vi "Edit.Path.TestLauncher.vi"() -> ()   [LabVIEW 2019, in "Edit.Path.lvclass"]
uses:
  Edit.Path.lvclass
  <vilib>/JKI/JKI SMO/SMO/Typedefs/SMOState --Enum.ctl
  C:/Program Files (x86)/National Instruments/LabVIEW 2019/vi.lib/JKI/JKI SMO/SMO/SMO.lvclass
  C:/Users/Albro/Documents/GitHub/AFM-Lithography/lvsrc/Classes/Subpanel/Edit/Edit/Edit.lvclass
  <vilib>/JKI/JKI SMO/SMO/SMO.lvclass/SMO.ctl
  <vilib>/JKI/JKI SMO/SMO/Private/ReftoDVR--SMO.vi
  <vilib>/JKI/JKI SMO/SMO/SMO.lvclass
  Edit/Edit.lvclass
panel:
  out "SMO State":T1
  out "error out":errorcluster
  in  "Stop":bool
  # "Basic SMO Test Launcher"
  # "For instructions on how to use the JKI State Machine Objects, examples and video tutorials, visit:\nhttp://jki.net/state-machine-objects/\n\nJKI State Machine Objects™\nhttp://jki.net/state-machine-objects/\nCopyright (C) 2005-2015, JKI <info@jki.net>\nALL RIGHTS RESERVED"
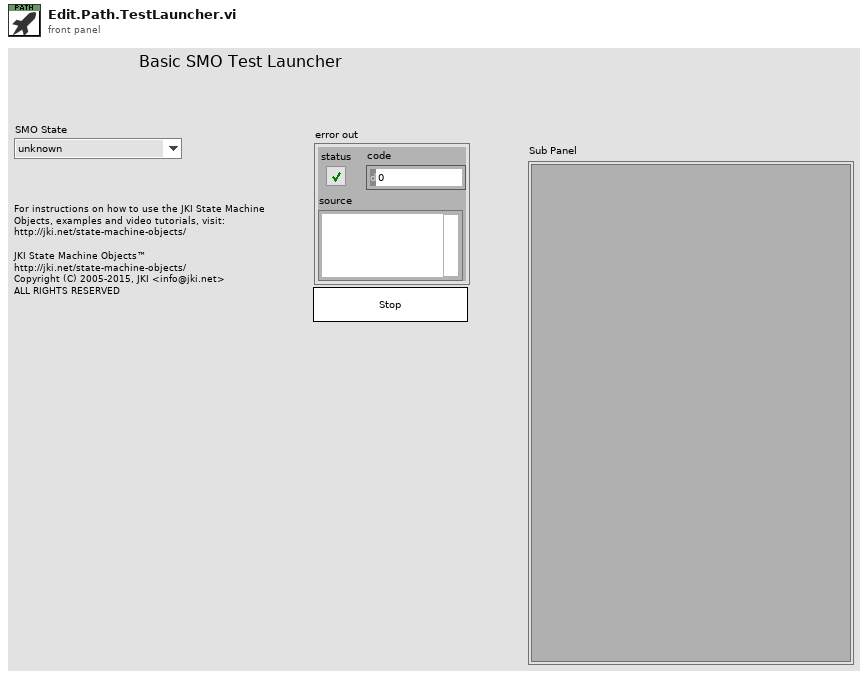
[diagram p1: front panel]
types:
  T1 = typedef "SMO.lvclass/SMOState --Enum.ctl" = enum16{"unknown", "Created", "Started", "Stopped"}
  T2 = typedef "SMO.lvclass/Public Events.ctl" = cluster{"Error":refnum<user-event>, "State":refnum<user-event>, "Reserve State":refnum<user-event>}
  T3 = cluster{"Event Registration Refnum":refnum<event-registration>}
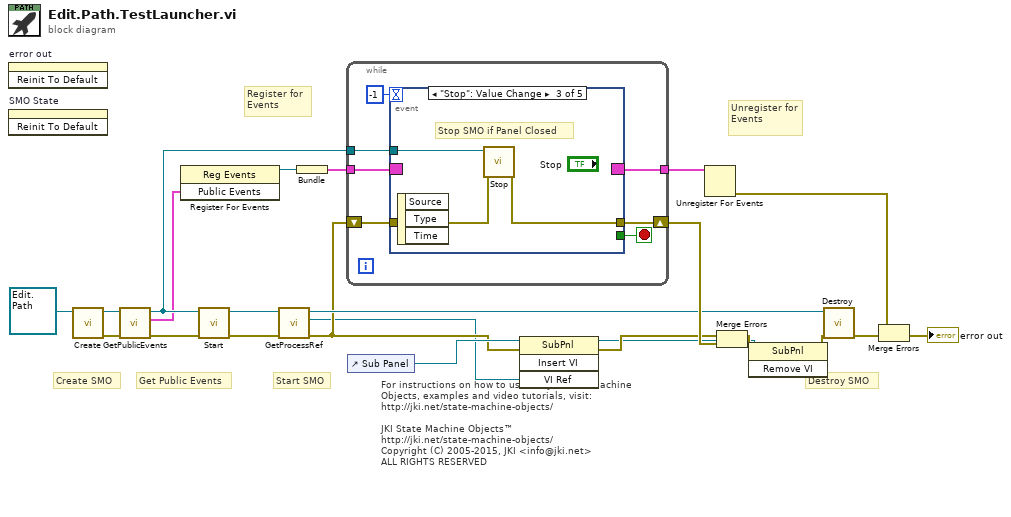
[diagram p0: block diagram]
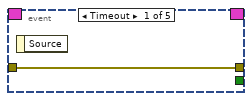
[diagram p2: hidden frame]
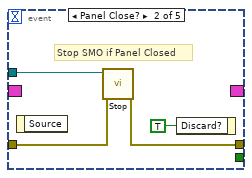
[diagram p3: hidden frame]
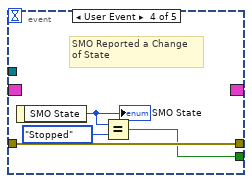
[diagram p4: hidden frame]
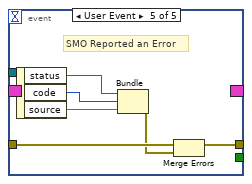
[diagram p5: hidden frame]
diagram:
  # "For instructions on how to use the JKI State Machine Objects, examples and video tutorials, visit:\nhttp://jki.net/state-machine-objects/\n\nJKI State Machine Objects™\nhttp://jki.net/state-machine-objects/\nCopyright (C) 2005-2015, JKI <info@jki.net>\nALL RIGHTS RESERVED"
  # "Get Public Events"
  # "Start SMO"
  # "Destroy SMO"
  # "Create SMO"
  # "Unregister for Events"
  # "Register for Events"
  n1 = invoke on="error out" class="Clust (strict)" method="Reinit To Default"() -> ()  [unwired: 3 in, 3 out]
  n2 = invoke on="SMO State" class="Enum (strict)" method="Reinit To Default"() -> ()  [unwired: 3 in, 3 out]
  n3 = call <vilib>:"Create.vi"("SMO"=refnum<class "Edit.Path.lvclass"> refnum ("SMO.Template.lvclass")) -> ("error out"=w15:errorcluster, "SMO out"=w16:refnum<class "Edit.Path.lvclass">)  [unwired: 8 in, 1 out]
  n4 = call <vilib>:"GetPublicEvents.vi"("error in (no error)"=w15, "SMO"=w16) -> ("error out"=w14:errorcluster, "Public Events"=w12:T2, "SMO out"=w13:refnum<class "Edit.Path.lvclass">)  [unwired: 7 in]
  n5 = register-events(w12) -> (reference out=w11:refnum<event-registration>)  [unwired: 2 in, 1 out]
  n6 = call <vilib>:"Start.vi"("error in (no error)"=w14, "SMO"=w13) -> ("error out"=w4:errorcluster, "SMO out"=w6:refnum<class "Edit.Path.lvclass">)  [unwired: 8 in]
  n7 = call "GetProcessRef.vi"("error in (no error)"=w4, "Edit in"=w6) -> ("error out"=w3:errorcluster, "Static VI Ref"=w2:refnum<vi>, "Edit out"=w5:refnum<class "Edit.Path.lvclass">)  [unwired: 7 in]
  n8 = Bundle("Event Registration Refnum"=w11) -> (w22:T3)  [unwired: 1 in]
  n9 = while {
    shift-right: [w29] -> w21
    shift-left: w3 -> [w28]
    tunnel: w22 -> [w27]
    tunnel: [w26] -> w23
    tunnel: w13 -> [w25]
    stop <- w30 stop-if-true
    n10 = event shown="[2] \"Stop\": Value Change" {
      selector: w27 -> [_ _ _ _ _]
      dyn-events: [_ _ _ _ _] -> w26
      timeout: -1 -> [_ _ _ _ _]
      tunnel: [_ _ _ w39 _] -> w30
      tunnel: w25 -> [_ w35 w38 _ _]
      tunnel: [w31 w34 w37 w42 w46] -> w29
      tunnel: w28 -> [w31 w33 w36 w42 w44]
      event Timeout {
        n11 = event-data() -> ()  [unwired: 1 in, 1 out]
      }
      event Panel Close? {
        # "Stop SMO if Panel Closed"
        n12 = event-data() -> ()  [unwired: 1 in, 1 out]
        n13 = call <vilib>:"Stop.vi"("error in (no error)"=w33, "SMO"=w35) -> ("error out"=w34:errorcluster)  [unwired: 8 in, 1 out]
        n14 = event-data("Discard?"=TRUE ("OK")) -> ()  [unwired: 1 in, 1 out]
      }
      event "Stop": Value Change {
        # "Stop SMO if Panel Closed"
        n15 = event-data() -> ()  [unwired: 1 in, 3 out]
        n16 = call <vilib>:"Stop.vi"("error in (no error)"=w36, "SMO"=w38) -> ("error out"=w37:errorcluster)  [unwired: 8 in, 1 out]
      }
      event User Event {
        # "SMO Reported a Change\nof State"
        n17 = event-data() -> ("SMO State"=w41:T1)  [unwired: 1 in]
        "SMO State" <- w41
        n18 = Equal?(x=w41, y=SMOState_--Enum."Stopped") -> (x = y?=w39:bool)
      }
      event User Event {
        # "SMO Reported an Error"
        n19 = event-data() -> ("status"=w45:bool, "code"=w48:i32, "source"=w47:string)  [unwired: 1 in]
        n20 = Bundle("status"=w45, "code"=w48, "source"=w47) -> (w43:errorcluster)  [unwired: 1 in]
        n21 = Merge Errors(w44, w43) -> (w46:errorcluster)
      }
    }
  }
  n22 = control-ref of="Sub Panel"() -> (w10:refnum<vi>)
  n23 = invoke class="SubPnl" method="Insert VI"(reference=w10, error in=w3, "VI Ref"=w2) -> (reference out=w1:refnum<vi>, error out=w7:errorcluster)  [unwired: 1 in, 2 out]
  n24 = Unregister For Events(event registration refnum=w23) -> (error out=w20:errorcluster)  [unwired: 1 in]
  n25 = Merge Errors(w7, w21) -> (w9:errorcluster)
  n26 = invoke class="SubPnl" method="Remove VI"(reference=w1, error in=w9) -> (error out=w8:errorcluster)  [unwired: 1 in, 2 out]
  n27 = call <vilib>:"Destroy.vi"("error in (no error)"=w8, "SMO"=w5) -> ("error out"=w18:errorcluster)  [unwired: 9 in]
  n28 = Merge Errors(w20, w18) -> (→"error out":errorcluster)
